vi "NISE.local.Close Session.vi"(0 "SLSC Local in":refnum<class "SLSC Interface.lvclass">, 11 "error in (no error)":errorcluster) -> (15 "error out":errorcluster)   [LabVIEW 2016, in "SLSC Interface.lvclass"]
uses:
  SLSC Interface Class/SLSC Interface.lvclass
  SLSC Interface Class/NISE.Read session.vi
  <vilib>/SLSC/Close Session.vi
  <vilib>/SLSC/SLSC.lvlib
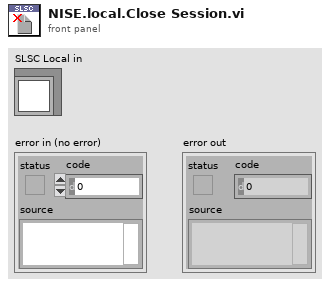
[diagram p1: front panel]
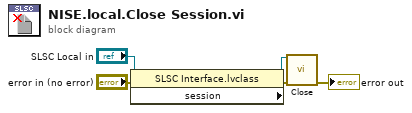
[diagram p0: block diagram]
diagram:
  n1 = property class="SLSC Interface.lvclass"(reference="SLSC Local in", error in="error in (no error)") -> (error out=w3:errorcluster, "session"=w2:refnum<k21>)  [unwired: 1 out]
  n2 = call-poly <vilib>:"Close.vi"("session in"=w2, "error in (no error)"=w3) -> ("error out"=→"error out":errorcluster)  [unwired: 13 in]
